vi "log_acquisition.vi"(1 "log_data":T1) -> (0 "Log":string)   [LabVIEW 2016]
uses:
  log_data.ctl
  log_status.ctl
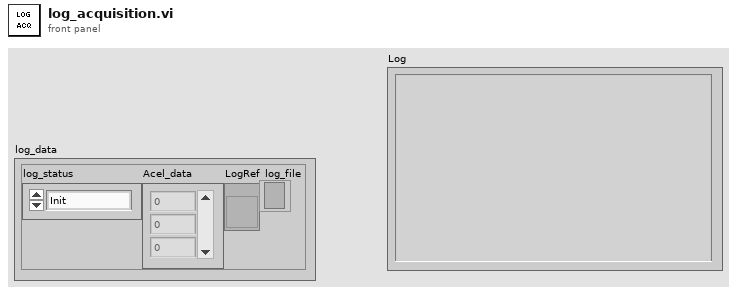
[diagram p1: front panel]
types:
  T1 = typedef "log_data.ctl" = cluster{"log_status":T2, "Acel_data":dbl[], "LogRef":refnum<vi>, "log_file":refnum<file>}
  T2 = typedef "log_status.ctl" = enum16{"Init", "Ready", "Config", "Running", "Error", "End"}
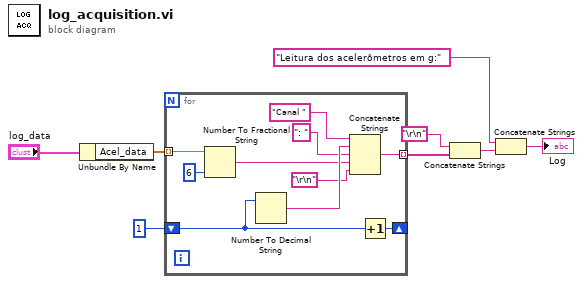
[diagram p0: block diagram]
diagram:
  n1 = Unbundle By Name("log_data") -> ("Acel_data"=w1:dbl[])
  n2 = for {
    tunnel: w1 -> [w18] mode=indexing
    shift-right: [w16] -> _
    shift-left: i16 1 ("precision (6)") -> [w15]
    tunnel: [w10] -> w3 mode=indexing
    n3 = Number To Fractional String(number=w18, precision (6)=i16 6) -> (F-format string=w11:string)  [unwired: 2 in]
    n4 = Number To Decimal String(number=w15) -> (decimal integer string=w14:string)  [unwired: 1 in]
    n5 = Concatenate Strings("Canal " ("string"), w14, ": " ("string"), w11, "\r\n") -> (w10:string)
    n6 = Increment(x=w15) -> (x+1=w16:i16)
  }
  n7 = Concatenate Strings("\r\n", w3) -> (w7:string)
  n8 = Concatenate Strings("Leitura dos acelerômetros em g:" ("string"), w7) -> (→"Log":string)
